vi "Initialize.vi"(6 "optional":variant, 8 "error in (no error)":errorcluster, 11 "Structure in":refnum<class "Structure.lvclass">) -> (0 "error out":errorcluster, 3 "Structure out":refnum<class "Structure.lvclass">)   [LabVIEW 2009, in "Structure.lvclass"]
uses:
  Structure.lvclass
  Structure.lvclass/Structure.ctl
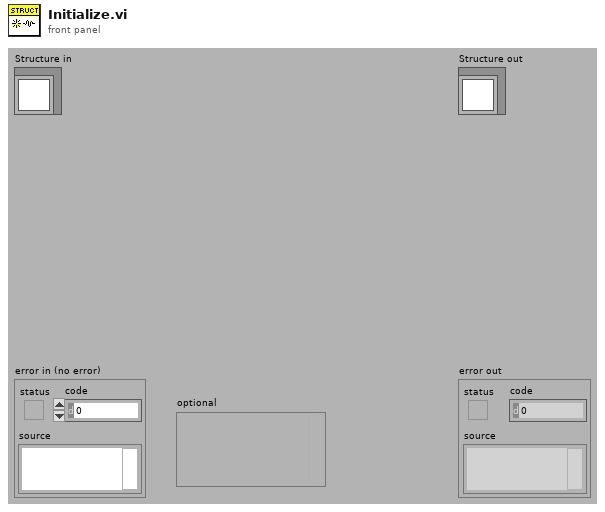
[diagram p1: front panel]
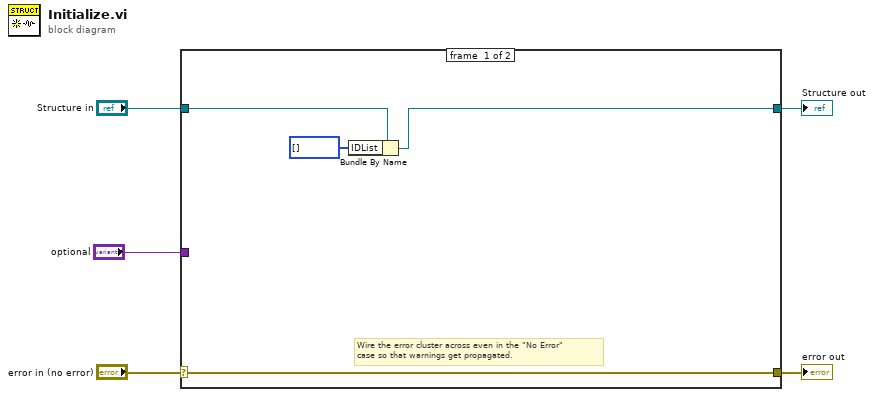
[diagram p0: block diagram]
diagram:
  n1 = case shown="No Error" "error in (no error)" {
    selector: "error in (no error)" -> [w9 w11]
    tunnel: [w9 w11] -> w4
    tunnel: [w7 w10] -> w2
    tunnel: "Structure in" -> [w8 w10]
    tunnel: "optional" -> [_ _]
    frame #0 {
      # "Wire the error cluster across even in the \"No Error\"\ncase so that warnings get propagated."
      n2 = Bundle By Name(cluster=w8, "IDList"=u32[] []) -> (w7:refnum<class "Structure.lvclass">)
    }
    frame #1 {
    }
  }
  "error out" <- w4
  "Structure out" <- w2
